vi "UI_(08A)_Prepare_loaded_data_playback.vi"(4 "Timeline max, s":dbl, 6 "error in (no error)":errorcluster, 8 "Timeline min, s":dbl, 9 "Settings cluster in":T1={"Defaults"={"Default User"=0.0, "VISA Resource Name "=""}, "Recording and saving"={"Researcher name"="", "Name prefix"="", "Data post-processing"={"Filter type"=enum."Savitzky-Golay", "Length"=31, "Order"=3}, "Stop at"=0.0, "\"Stop at\" enabled"=FALSE, "Default save folder path"=path "", "Acquisition FPS"=enum."Max"}, "Geometry"={"Cage diameter, mm"=0, "Starting angle MIDFIELD"=0, "Starting angle BORDER"=0, "Radius, mm CENTER"=0, "Radius, mm MIDFIELD"=0, "N segments MIDFIELD"=0, "N segments BORDER"=0, "R-gap, mm"=0.0, "Bridge swap"=FALSE, "Bridge H. offset"=0.0, "Bridge V. offset"=0.0, "Twisted neck"=FALSE, "Alt. magn. orientation"=FALSE, "Sensor board size"=enum."Small"}, "IO parameters"={"IO general config."=0, "IO 1 configuration"=0, "IO 2 configuration"=0, "IO 3 configuration"=0, "IO 4 configuration"=0, "Activate ext. RS-232"=0, "IO inversion config."=0, "Sync capability"=1}, "Stimulus presets array"=[{"Event type"=0, "Dur., s"=0.0, "Stim., s"=0.0, "TTL out N"=1, "Set/Clear"=FALSE, "Stim. has been set"=FALSE}, {"Event type"=0, "Dur., s"=0.0, "Stim., s"=0.0, "TTL out N"=1, "Set/Clear"=FALSE, "Stim. has been set"=FALSE}, {"Event type"=0, "Dur., s"=0.0, "Stim., s"=0.0, "TTL out N"=1, "Set/Clear"=FALSE, "Stim. has been set"=FALSE}, {"Event type"=0, "Dur., s"=0.0, "Stim., s"=0.0, "TTL out N"=1, "Set/Clear"=FALSE, "Stim. has been set"=FALSE}, {"Event type"=0, "Dur., s"=0.0, "Stim., s"=0.0, "TTL out N"=1, "Set/Clear"=FALSE, "Stim. has been set"=FALSE}, {"Event type"=0, "Dur., s"=0.0, "Stim., s"=0.0, "TTL out N"=1, "Set/Clear"=FALSE, "Stim. has been set"=FALSE}, {"Event type"=0, "Dur., s"=0.0, "Stim., s"=0.0, "TTL out N"=1, "Set/Clear"=FALSE, "Stim. has been set"=FALSE}, {"Event type"=0, "Dur., s"=0.0, "Stim., s"=0.0, "TTL out N"=1, "Set/Clear"=FALSE, "Stim. has been set"=FALSE}, {"Event type"=0, "Dur., s"=0.0, "Stim., s"=0.0, "TTL out N"=1, "Set/Clear"=FALSE, "Stim. has been set"=FALSE}, {"Event type"=0, "Dur., s"=0.0, "Stim., s"=0.0, "TTL out N"=1, "Set/Clear"=FALSE, "Stim. has been set"=FALSE}, {"Event type"=0, "Dur., s"=0.0, "Stim., s"=0.0, "TTL out N"=1, "Set/Clear"=FALSE, "Stim. has been set"=FALSE}, {"Event type"=0, "Dur., s"=0.0, "Stim., s"=0.0, "TTL out N"=1, "Set/Clear"=FALSE, "Stim. has been set"=FALSE}, {"Event type"=0, "Dur., s"=0.0, "Stim., s"=0.0, "TTL out N"=1, "Set/Clear"=FALSE, "Stim. has been set"=FALSE}, {"Event type"=0, "Dur., s"=0.0, "Stim., s"=0.0, "TTL out N"=1, "Set/Clear"=FALSE, "Stim. has been set"=FALSE}], "Calibration parameters"={"Timing calibration sw/hw"=1.0, "True FPS"=80.0, "True frame time, s"=0.0125, "Disp. calibration info"=[]}, "Settings loaded OK"=FALSE} {"Calibration parameters"."True frame time, s" format="%.10g"; "Calibration parameters"."Disp. calibration info"."Speed, µl per ms" format="%.3g"; "Calibration parameters"."True FPS" format="%.10g"; "Calibration parameters"."Timing calibration sw/hw" format="%.10g"; "Stimulus presets array"."Event type" items=["Stay for N seconds"]; "Stimulus presets array"."TTL out N" items=["1"=1, "2"=2, "1+2"=3]; "Recording and saving"."Data post-processing"."Order" min=3 max=11 step=2; "Recording and saving"."Data post-processing"."Length" min=5 max=301 step=2; "Geometry"."Cage diameter, mm" scale=0.0..340.0}, 10 "All references in":T11) -> (0 "error out":errorcluster, 2 "Settings cluster out":T1={"Defaults"={"Default User"=0.0, "VISA Resource Name "=""}, "Recording and saving"={"Researcher name"="", "Name prefix"="", "Data post-processing"={"Filter type"=enum."Savitzky-Golay", "Length"=31, "Order"=3}, "Stop at"=0.0, "\"Stop at\" enabled"=FALSE, "Default save folder path"=path "", "Acquisition FPS"=enum."Max"}, "Geometry"={"Cage diameter, mm"=0, "Starting angle MIDFIELD"=0, "Starting angle BORDER"=0, "Radius, mm CENTER"=0, "Radius, mm MIDFIELD"=0, "N segments MIDFIELD"=0, "N segments BORDER"=0, "R-gap, mm"=0.0, "Bridge swap"=FALSE, "Bridge H. offset"=0.0, "Bridge V. offset"=0.0, "Twisted neck"=FALSE, "Alt. magn. orientation"=FALSE, "Sensor board size"=enum."Small"}, "IO parameters"={"IO general config."=0, "IO 1 configuration"=0, "IO 2 configuration"=0, "IO 3 configuration"=0, "IO 4 configuration"=0, "Activate ext. RS-232"=0, "IO inversion config."=0, "Sync capability"=1}, "Stimulus presets array"=[{"Event type"=0, "Dur., s"=0.0, "Stim., s"=0.0, "TTL out N"=1, "Set/Clear"=FALSE, "Stim. has been set"=FALSE}, {"Event type"=0, "Dur., s"=0.0, "Stim., s"=0.0, "TTL out N"=1, "Set/Clear"=FALSE, "Stim. has been set"=FALSE}, {"Event type"=0, "Dur., s"=0.0, "Stim., s"=0.0, "TTL out N"=1, "Set/Clear"=FALSE, "Stim. has been set"=FALSE}, {"Event type"=0, "Dur., s"=0.0, "Stim., s"=0.0, "TTL out N"=1, "Set/Clear"=FALSE, "Stim. has been set"=FALSE}, {"Event type"=0, "Dur., s"=0.0, "Stim., s"=0.0, "TTL out N"=1, "Set/Clear"=FALSE, "Stim. has been set"=FALSE}, {"Event type"=0, "Dur., s"=0.0, "Stim., s"=0.0, "TTL out N"=1, "Set/Clear"=FALSE, "Stim. has been set"=FALSE}, {"Event type"=0, "Dur., s"=0.0, "Stim., s"=0.0, "TTL out N"=1, "Set/Clear"=FALSE, "Stim. has been set"=FALSE}, {"Event type"=0, "Dur., s"=0.0, "Stim., s"=0.0, "TTL out N"=1, "Set/Clear"=FALSE, "Stim. has been set"=FALSE}, {"Event type"=0, "Dur., s"=0.0, "Stim., s"=0.0, "TTL out N"=1, "Set/Clear"=FALSE, "Stim. has been set"=FALSE}, {"Event type"=0, "Dur., s"=0.0, "Stim., s"=0.0, "TTL out N"=1, "Set/Clear"=FALSE, "Stim. has been set"=FALSE}, {"Event type"=0, "Dur., s"=0.0, "Stim., s"=0.0, "TTL out N"=1, "Set/Clear"=FALSE, "Stim. has been set"=FALSE}, {"Event type"=0, "Dur., s"=0.0, "Stim., s"=0.0, "TTL out N"=1, "Set/Clear"=FALSE, "Stim. has been set"=FALSE}, {"Event type"=0, "Dur., s"=0.0, "Stim., s"=0.0, "TTL out N"=1, "Set/Clear"=FALSE, "Stim. has been set"=FALSE}, {"Event type"=0, "Dur., s"=0.0, "Stim., s"=0.0, "TTL out N"=1, "Set/Clear"=FALSE, "Stim. has been set"=FALSE}], "Calibration parameters"={"Timing calibration sw/hw"=1.0, "True FPS"=80.0, "True frame time, s"=0.0125, "Disp. calibration info"=[]}, "Settings loaded OK"=FALSE} {"Calibration parameters"."True frame time, s" format="%.10g"; "Calibration parameters"."Disp. calibration info"."Speed, µl per ms" format="%.3g"; "Calibration parameters"."True FPS" format="%.10g"; "Calibration parameters"."Timing calibration sw/hw" format="%.10g"; "Stimulus presets array"."Event type" items=["Stay for N seconds"]; "Stimulus presets array"."TTL out N" items=["1"=1, "2"=2, "1+2"=3]; "Recording and saving"."Data post-processing"."Order" min=3 max=11 step=2; "Recording and saving"."Data post-processing"."Length" min=5 max=301 step=2; "Geometry"."Cage diameter, mm" scale=0.0..340.0}, 3 "All references out":T11)   [LabVIEW 2018, in "Tracker.lvlib"]
uses:
  Tracker.lvlib
  Controls/CTL_All_References.ctl
  Controls/CTL_Controls_References.ctl
  Controls/CTL_Indicators_References.ctl
  Controls/CTL_Panes_and_VIs_References.ctl
  Controls/CTL_Histogram_Properties.ctl
  <vilib>/Utility/miscctls.llb/LVRangeTypeDef.ctl
  Controls/CTL_Settings_cluster.ctl
  Controls/CTL_Filter_selector.ctl
  Controls/CTL_Acquisition_speed_selector.ctl
  Controls/CTL_Segmented_plot_parameters.ctl
  Controls/CTL_IO_params_cluster.ctl
  Controls/CTL_Single_stimulus_setting.ctl
  Controls/CTL_Calibration_parameters.ctl
  Controls/CTL_Dispenser_calibration_info.ctl
  <vilib>/Utility/error.llb/Error Cluster From Error Code.vi
  <vilib>/ErrorRing/Error Ring.xnode
panel:
  in  "Histogram initialization cluster":T9={"X Scale.Range"={"Minimum"=0.0, "Maximum"=13.0, "Increment"=1.0, "Minor Increment"=1.0, "Start"=0.0}, "Caption.Text"="Zone preference (normalized)", "X Scale.Offset and Multiplier:Multiplier"=1.0, "X Scale.Offset and Multiplier:Offset"=0.0, "X Scale.Scale Fit"=2, "X Scale.Display Format:Precision"=0, "Y Scale.Mapping Mode"=0, "Zones preference empty initialized array"=[0, 0, 0, 0, 0, 0, 0, 0, 0, 0, 0, 0, 0, 0], "Plot.Fill/Point Color"=15790320}
  out "Panes references":T14
  out "Controls references params":string[][](array[string])
  out "Indicators references params":string[][](array[string])
  out "Indicators references":T13
  out "Controls references":T12
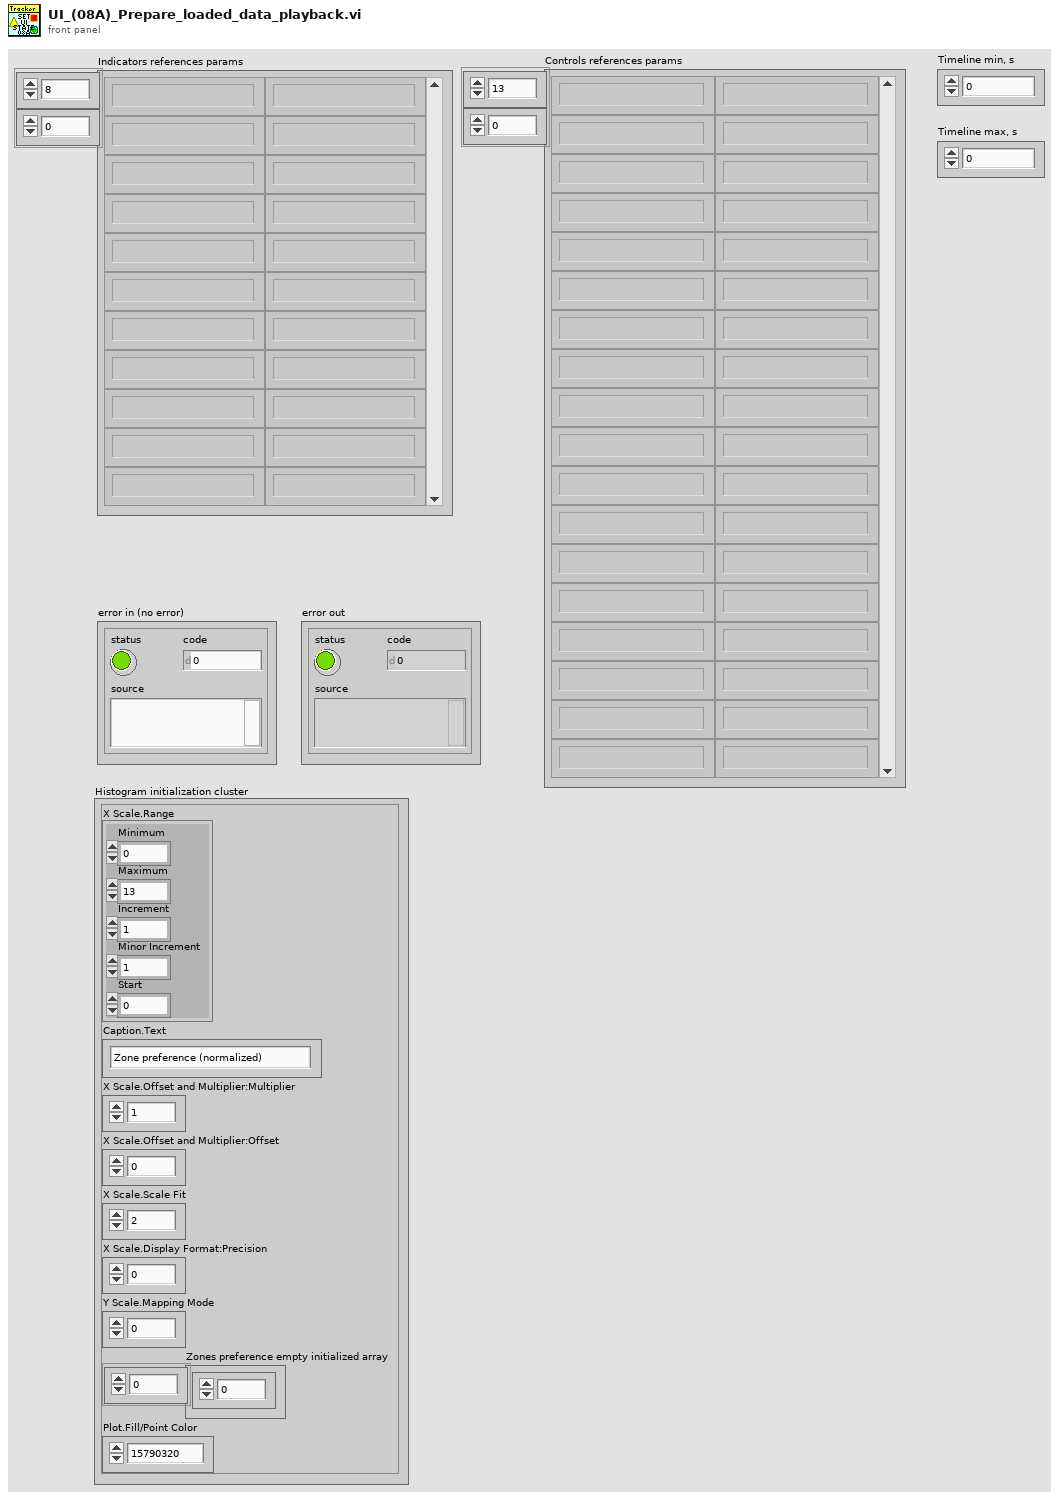
[diagram p1: front panel]
types:
  T1 = typedef "Tracker.lvlib/CTL_Settings_cluster.ctl" = cluster{"Defaults":cluster{"Default User":dbl, "VISA Resource Name ":string}, "Recording and saving":cluster{"Researcher name":string, "Name prefix":string, "Data post-processing":T2, "Stop at":dbl, "\"Stop at\" enabled":bool, "Default save folder path":path, "Acquisition FPS":T3}, "Geometry":T4, "IO parameters":T5, "Stimulus presets array":T6[], "Calibration parameters":T7, "Settings loaded OK":bool}
  T2 = typedef "Tracker.lvlib/CTL_Filter_selector.ctl" = cluster{"Filter type":enum16{"None", "Savitzky-Golay"}, "Length":i32, "Order":i32}
  T3 = typedef "Tracker.lvlib/CTL_Acquisition_speed_selector.ctl" = enum16{"Max", "Optimal", "Eco"}
  T4 = typedef "Tracker.lvlib/CTL_Segmented_plot_parameters.ctl" = cluster{"Cage diameter, mm":u16, "Starting angle MIDFIELD":i16, "Starting angle BORDER":i16, "Radius, mm CENTER":u16, "Radius, mm MIDFIELD":u16, "N segments MIDFIELD":u8, "N segments BORDER":u8, "R-gap, mm":sgl, "Bridge swap":bool, "Bridge H. offset":sgl, "Bridge V. offset":sgl, "Twisted neck":bool, "Alt. magn. orientation":bool, "Sensor board size":enum16{"Small", "Large"}}
  T5 = typedef "Tracker.lvlib/CTL_IO_params_cluster.ctl" = cluster{"IO general config.":u16, "IO 1 configuration":u16, "IO 2 configuration":u16, "IO 3 configuration":u16, "IO 4 configuration":u16, "Activate ext. RS-232":u16, "IO inversion config.":u16, "Sync capability":u8}
  T6 = typedef "Tracker.lvlib/CTL_Single_stimulus_setting.ctl" = cluster{"Event type":u16, "Dur., s":sgl, "Stim., s":sgl, "TTL out N":u16, "Set/Clear":bool, "Stim. has been set":bool}
  T7 = typedef "Tracker.lvlib/CTL_Calibration_parameters.ctl" = cluster{"Timing calibration sw/hw":dbl, "True FPS":dbl, "True frame time, s":dbl, "Disp. calibration info":T8}
  T8 = typedef "Tracker.lvlib/CTL_Dispenser_calibration_info.ctl" = cluster{"Channel":u8, "Speed, µl per ms":dbl}[]
  T9 = typedef "Tracker.lvlib/CTL_Histogram_Properties.ctl" = cluster{"X Scale.Range":T10, "Caption.Text":string, "X Scale.Offset and Multiplier:Multiplier":dbl, "X Scale.Offset and Multiplier:Offset":dbl, "X Scale.Scale Fit":u8, "X Scale.Display Format:Precision":u8, "Y Scale.Mapping Mode":u8, "Zones preference empty initialized array":i32[], "Plot.Fill/Point Color":u32}
  T10 = typedef "LVRangeTypeDef.ctl" = cluster{"Minimum":dbl, "Maximum":dbl, "Increment":dbl, "Minor Increment":dbl, "Start":dbl}
  T11 = typedef "Tracker.lvlib/CTL_All_References.ctl" = cluster{"Controls references":T12, "Indicators references":T13, "Service references":T14}
  T12 = typedef "Tracker.lvlib/CTL_Controls_References.ctl" = cluster{"Check HW connection":refnum<vi>, "Save settings":refnum<vi>, "Reset zones":refnum<vi>, "Reset stimuli":refnum<vi>, "Record/Stop":refnum<vi>, "Reset barplot":refnum<vi>, "Multiplyer of chart RX":refnum<vi>, "Show zones":refnum<vi>, "Show magnets":refnum<vi>, "Show heatmap":refnum<vi>, "Show full track":refnum<vi>, "Open File":refnum<vi>, "Play/Pause":refnum<vi>, "Trace, s":refnum<vi>, "Playback speed":refnum<vi>, "Timeline":refnum<vi>, "By Zone stim. setup":refnum<vi>, "Set/Rec and Analyse Tab":refnum<vi>, "Cage radial segmentation":refnum<vi>, "Set IO config":refnum<vi>, "Rainbow (time)":refnum<vi>, "Rainbow (speed)":refnum<vi>}
  T13 = typedef "Tracker.lvlib/CTL_Indicators_References.ctl" = cluster{"HW info":refnum<vi>, "Port":refnum<vi>, "Ready":refnum<vi>, "IO status indicator":refnum<vi>, "Current Time":refnum<vi>, "Record timestamp":refnum<vi>, "Mouse speed":refnum<vi>, "Mouse speed, mm/s":refnum<vi>, "Running, perc. of time":refnum<vi>, "Histograms":refnum<vi>, "Cage size":refnum<vi>}
  T14 = typedef "Tracker.lvlib/CTL_Panes_and_VIs_References.ctl" = cluster{"Pane":refnum<vi>, "This VI":refnum<vi>, "Menu":refnum<k9>}
  T15 = enum8{"Enabled", "Disabled", "Disabled and Grayed Out"}
  T16 = cluster{"Slider":dbl, "Slider":dbl, "Slider":dbl}
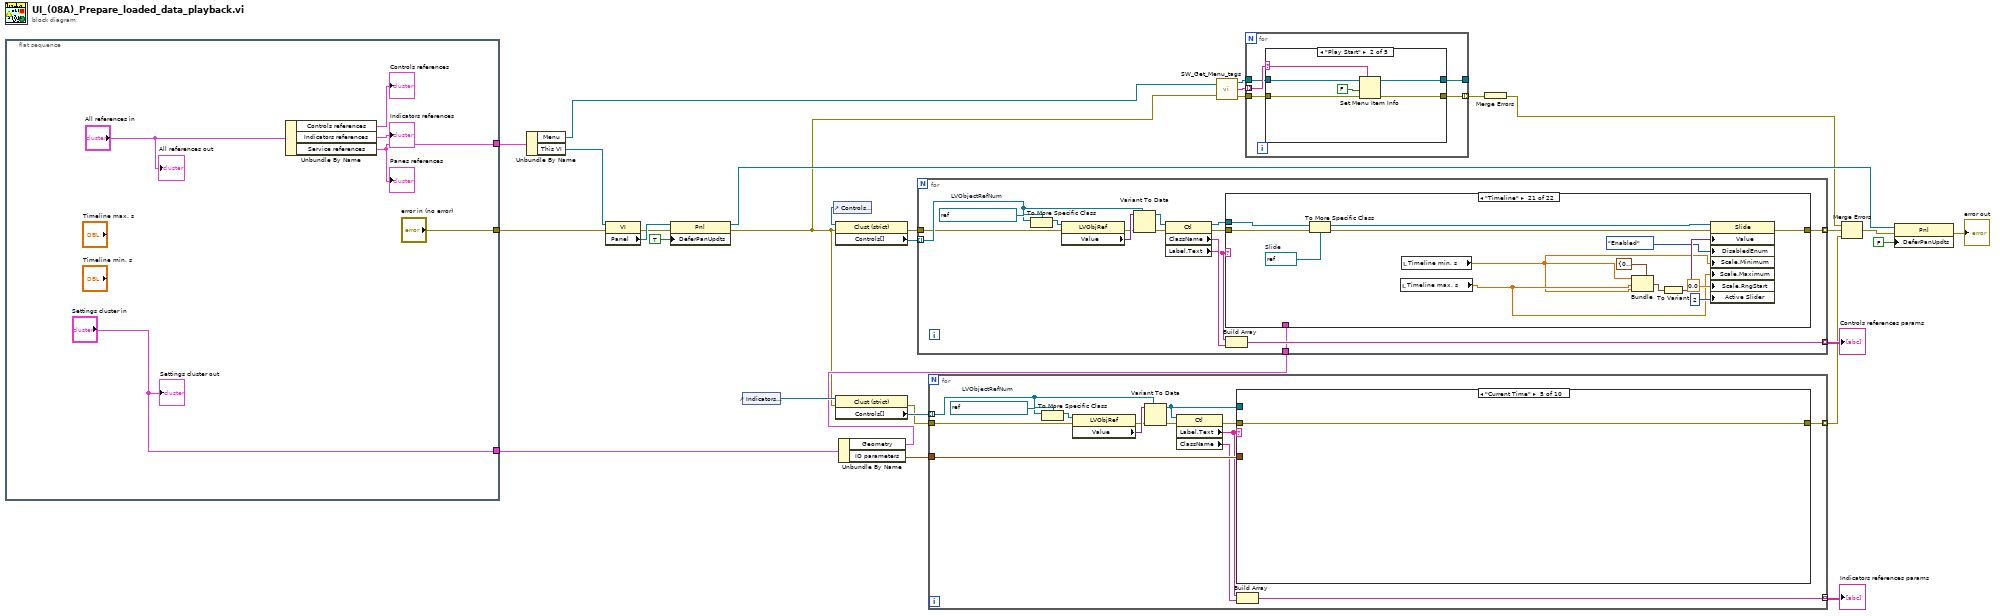
[diagram p0: block diagram]
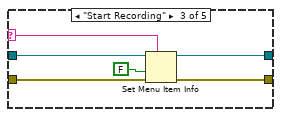
[diagram p3: hidden frame]
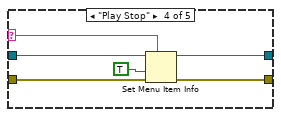
[diagram p4: hidden frame]
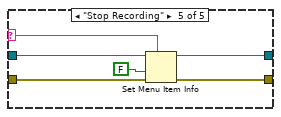
[diagram p5: hidden frame]
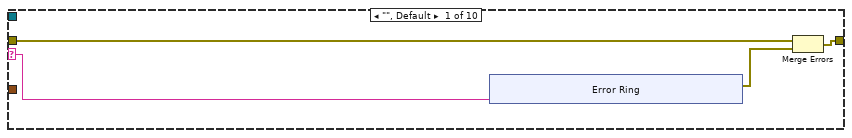
[diagram p6: hidden frame]
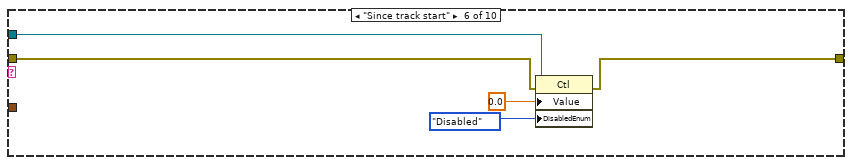
[diagram p10: hidden frame]
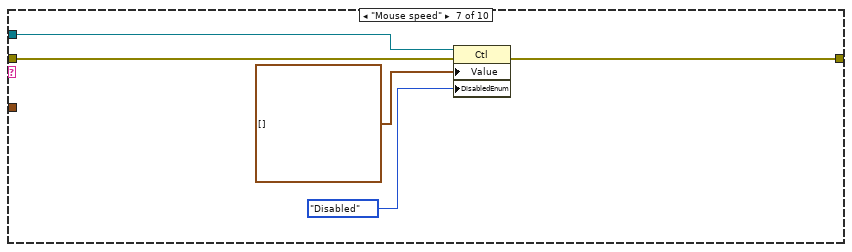
[diagram p11: hidden frame]
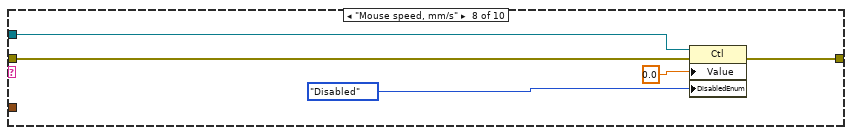
[diagram p12: hidden frame]
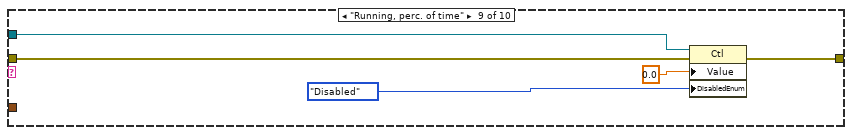
[diagram p13: hidden frame]
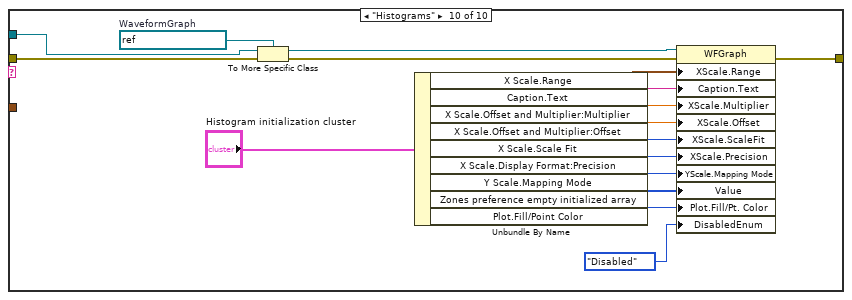
[diagram p14: hidden frame]
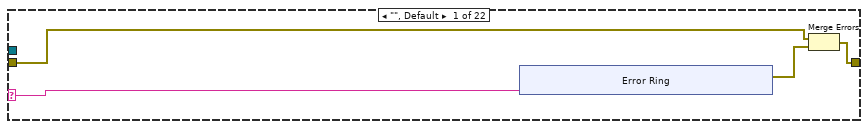
[diagram p15: hidden frame]
diagram:
  n1 = flat-sequence {
    tunnel: [w33] -> w24
    tunnel: ["Settings cluster in"] -> w11
    tunnel: ["error in (no error)"] -> w9
    frame #0 {
      n2 = Unbundle By Name("All references in") -> ("Controls references"=→"Controls references":T12, "Indicators references"=→"Indicators references":T13, "Service references"=w33:T14)
      "Panes references" <- w33
      "All references out" <- "All references in"
      "Settings cluster out" <- "Settings cluster in"
    }
  }
  n3 = Unbundle By Name(w24) -> ("Menu"=w3:refnum<k9>, "This VI"=w21:refnum<vi>)
  n4 = property class="VI"(reference=w21, error in=w9) -> (error out=w14:errorcluster, "Panel"=w23:refnum<vi>)  [unwired: 1 out]
  n5 = property class="Pnl"(reference=w23, error in=w14, "DeferPanUpdts"=TRUE ("Defer Panel Updates")) -> (reference out=w15:refnum<vi>, error out=w2:errorcluster)
  n6 = control-ref of="Indicators references"() -> (w27:refnum<vi>)
  n7 = control-ref of="Controls references"() -> (w29:refnum<vi>)
  n8 = property class="Clust (strict)"(reference=w29, error in=w2) -> (error out=w20:errorcluster, "Controls[]"=w30:refnum<vi>[])  [unwired: 1 out]
  n9 = property class="Clust (strict)"(reference=w27, error in=w2) -> (error out=w19:errorcluster, "Controls[]"=w28:refnum<vi>[])  [unwired: 1 out]
  n10 = Unbundle By Name(w11) -> ("Geometry"=w8:T4, "IO parameters"=w10:T5)
  n11 = for {
    tunnel: w30 -> [w48] mode=indexing
    tunnel: [w45] -> w25 mode=indexing
    tunnel: w20 -> [w44]
    tunnel: [w40] -> w12 mode=indexing
    tunnel: w8 -> [w37]
    w50 = refnum<vi> refnum  # LVObjectRefNum
    n12 = To More Specific Class(target class=w50, reference=w48) -> (specific class reference=w51:refnum<vi>)  [unwired: 1 in, 1 out]
    n13 = property class="LVObjRef"(reference=w51, error in=w44) -> (error out=w43:errorcluster, "Value"=w49:variant)  [unwired: 1 out]
    n14 = Variant To Data(error in=w43, type=w48, Variant=w49) -> (data=w47:refnum<vi>, error out=w42:errorcluster)
    n15 = property class="Ctl"(reference=w47, error in=w42) -> (reference out=w38:refnum<vi>, error out=w39:errorcluster, "ClassName"=w46:string, "Label.Text"=w41:string)
    n16 = case shown="\"Timeline\"" w41 {
      selector: w41 -> [w52 _ _ _ _ _ _ _ _ _ _ _ _ _ _ _ _ _ _ _ _ _]
      tunnel: [w54 w63 w64 w65 w66 w67 w68 w69 w72 w80 w88 w96 w102 w103 w112 w118 w128 w129 w132 w140 w154 w160] -> w40
      tunnel: w39 -> [w55 w63 w64 w65 w66 w67 w68 w69 w74 w82 w90 w98 w102 w105 w114 w118 w128 w129 w134 w142 w156 w160]
      tunnel: w38 -> [_ _ _ _ _ _ _ _ w77 w85 w93 w101 _ w104 w117 w119 _ _ w137 w145 w159 _]
      tunnel: w37 -> [_ _ _ _ _ _ _ _ _ _ _ _ _ _ _ _ _ _ _ _ _ _]
      frame "", Default {
        n17 = xnode "Error Ring"("parameter 0"=w52) -> ("error out"=w53:errorcluster)
        n18 = Merge Errors(w55, w53) -> (w54:errorcluster)
      }
      frame "Cage radial segmentation" {
      }
      frame "Set/Rec and Analyse Tab" {
      }
      frame "Check HW connection" {
      }
      frame "Save settings" {
      }
      frame "Set IO config" {
      }
      frame "Reset zones" {
      }
      frame "Reset stimuli" {
      }
      frame "Record/Stop" {
        w76 = refnum<vi> refnum  # Boolean
        n19 = To More Specific Class(target class=w76, reference=w77, error in=w74) -> (specific class reference=w75:refnum<vi>, error out=w73:errorcluster)
        n20 = property class="Bool"(reference=w75, error in=w73, "Value"=FALSE, "DisabledEnum"=T15."Disabled and Grayed Out" ("Disabled")) -> (error out=w72:errorcluster)  [unwired: 1 out]
      }
      frame "Reset barplot" {
        w84 = refnum<vi> refnum  # Boolean
        n21 = To More Specific Class(target class=w84, reference=w85, error in=w82) -> (specific class reference=w83:refnum<vi>, error out=w81:errorcluster)
        n22 = property class="Bool"(reference=w83, error in=w81, "Value"=FALSE, "DisabledEnum"=T15."Enabled" ("Disabled")) -> (error out=w80:errorcluster)  [unwired: 1 out]
      }
      frame "Multiplyer of chart RX" {
        w92 = refnum<vi> refnum  # Slide
        n23 = To More Specific Class(target class=w92, reference=w93, error in=w90) -> (specific class reference=w91:refnum<vi>, error out=w89:errorcluster)
        n24 = property class="Slide"(reference=w91, error in=w89, "Value"=u8 1, "DisabledEnum"=T15."Enabled" ("Disabled")) -> (error out=w88:errorcluster)  [unwired: 1 out]
      }
      frame "Show zones" {
        w100 = refnum<vi> refnum  # Boolean
        n25 = To More Specific Class(target class=w100, reference=w101, error in=w98) -> (specific class reference=w99:refnum<vi>, error out=w97:errorcluster)
        n26 = property class="Bool"(reference=w99, error in=w97, "Value"=TRUE, "DisabledEnum"=T15."Enabled" ("Disabled")) -> (error out=w96:errorcluster)  [unwired: 1 out]
      }
      frame "Show magnets" {
      }
      frame "Rainbow (speed)", "Rainbow (time)" {
        w106 = refnum<vi> refnum  # Boolean
        n27 = To More Specific Class(target class=w106, reference=w104, error in=w105) -> (specific class reference=w108:refnum<vi>, error out=w109:errorcluster)
        n28 = property class="Bool"(reference=w108, error in=w109, "DisabledEnum"=T15."Enabled" ("Disabled")) -> (error out=w103:errorcluster)  [unwired: 1 out]
      }
      frame "Show heatmap" {
        w116 = refnum<vi> refnum  # Boolean
        n29 = To More Specific Class(target class=w116, reference=w117, error in=w114) -> (specific class reference=w115:refnum<vi>, error out=w113:errorcluster)
        n30 = property class="Bool"(reference=w115, error in=w113, "Value"=FALSE, "DisabledEnum"=T15."Disabled and Grayed Out" ("Disabled")) -> (error out=w112:errorcluster)  [unwired: 1 out]
      }
      frame "Show full track" {
        n31 = disable-structure shown="Disabled" {
          disable-tunnel: w119 -> [w127 _]
          disable-tunnel: _ -> [w124 _]
          disable-tunnel: [w122 _] -> _
          frame Disabled {
            w126 = refnum<vi> refnum  # Boolean
            n32 = To More Specific Class(target class=w126, reference=w127, error in=w124) -> (specific class reference=w125:refnum<vi>, error out=w123:errorcluster)
            n33 = property class="Bool"(reference=w125, error in=w123, "Value"=FALSE, "DisabledEnum"=T15."Disabled and Grayed Out" ("Disabled")) -> (error out=w122:errorcluster)  [unwired: 1 out]
          }
          frame Enabled {
          }
        }
      }
      frame "Open File" {
      }
      frame "Play/Pause" {
      }
      frame "Trace, s" {
        w136 = refnum<vi> refnum  # Slide
        n34 = To More Specific Class(target class=w136, reference=w137, error in=w134) -> (specific class reference=w135:refnum<vi>, error out=w133:errorcluster)
        n35 = property class="Slide"(reference=w135, error in=w133, "Value"=u8 5, "DisabledEnum"=T15."Enabled" ("Disabled")) -> (error out=w132:errorcluster)  [unwired: 1 out]
      }
      frame "Playback speed" {
        w144 = refnum<vi> refnum  # Ring
        n36 = To More Specific Class(target class=w144, reference=w145, error in=w142) -> (specific class reference=w143:refnum<vi>, error out=w141:errorcluster)
        n37 = property class="Ring"(reference=w143, error in=w141, "Value"=u8 3, "DisabledEnum"=T15."Disabled and Grayed Out" ("Disabled")) -> (error out=w140:errorcluster)  [unwired: 1 out]
      }
      frame "Timeline" {
        w158 = refnum<vi> refnum  # Slide
        n38 = To More Specific Class(target class=w158, reference=w159, error in=w156) -> (specific class reference=w157:refnum<vi>, error out=w155:errorcluster)
        n39 = local read "Timeline max, s"() -> (w147:dbl)
        n40 = local read "Timeline min, s"() -> (w146:dbl)
        n41 = Bundle(cluster=T16 {"Slider"=0.0, "Slider"=0.0, "Slider"=0.0} ("Timeline"), "Slider"=w146, "Slider"=w147, "Slider"=w146) -> (w152:T16)
        n42 = To Variant(anything=w152) -> (Variant=w151:variant)
        n43 = property class="Slide"(reference=w157, error in=w155, "Value"=w151, "DisabledEnum"=T15."Enabled" ("Disabled"), "Scale.Minimum"=w146, "Scale.Maximum"=w147, "Scale.RngStart"=0.0 ("Scale.Range:Start"), "Active Slider"=2) -> (error out=w154:errorcluster)  [unwired: 1 out]
      }
      frame "By Zone stim. setup" {
      }
    }
    n44 = Build Array(w41, w46) -> (w45:string[])
  }
  "Controls references params" <- w25
  n45 = for {
    tunnel: w28 -> [w171] mode=indexing
    tunnel: [w161] -> w26 mode=indexing
    tunnel: w19 -> [w169]
    tunnel: [w165] -> w18 mode=indexing
    tunnel: w10 -> [w164]
    w173 = refnum<vi> refnum  # LVObjectRefNum
    n46 = To More Specific Class(target class=w173, reference=w171) -> (specific class reference=w174:refnum<vi>)  [unwired: 1 in, 1 out]
    n47 = property class="LVObjRef"(reference=w174, error in=w169) -> (error out=w168:errorcluster, "Value"=w172:variant)  [unwired: 1 out]
    n48 = Variant To Data(error in=w168, type=w171, Variant=w172) -> (data=w170:refnum<vi>, error out=w167:errorcluster)
    n49 = property class="Ctl"(reference=w170, error in=w167) -> (error out=w166:errorcluster, "Label.Text"=w163:string, "ClassName"=w162:string)  [unwired: 1 out]
    n50 = case shown="\"Current Time\"" w163 {
      selector: w163 -> [w175 _ _ _ _ _ _ _ _ _]
      tunnel: w170 -> [_ _ _ _ _ w190 w199 w204 w209 w226]
      tunnel: w166 -> [w178 w186 w187 w188 w189 w192 w198 w203 w208 w212]
      tunnel: [w177 w186 w187 w188 w189 w191 w197 w202 w207 w225] -> w165
      tunnel: w164 -> [_ _ _ _ _ _ _ _ _ _]
      frame "", Default {
        n51 = xnode "Error Ring"("parameter 0"=w175) -> ("error out"=w176:errorcluster)
        n52 = Merge Errors(w178, w176) -> (w177:errorcluster)
      }
      frame "Cage size", "HW info", "Port" {
      }
      frame "Ready" {
      }
      frame "IO status indicator" {
      }
      frame "Current Time" {
      }
      frame "Since track start" {
        n53 = property class="Ctl"(reference=w190, error in=w192, "Value"=0.0, "DisabledEnum"=T15."Disabled" ("Disabled")) -> (error out=w191:errorcluster)  [unwired: 1 out]
      }
      frame "Mouse speed" {
        n54 = property class="Ctl"(reference=w199, error in=w198, "Value"=waveform(dbl)[] [] ("History Data"), "DisabledEnum"=T15."Disabled" ("Disabled")) -> (error out=w197:errorcluster)  [unwired: 1 out]
      }
      frame "Mouse speed, mm/s" {
        n55 = property class="Ctl"(reference=w204, error in=w203, "Value"=0.0, "DisabledEnum"=T15."Disabled" ("Disabled")) -> (error out=w202:errorcluster)  [unwired: 1 out]
      }
      frame "Running, perc. of time" {
        n56 = property class="Ctl"(reference=w209, error in=w208, "Value"=0.0, "DisabledEnum"=T15."Disabled" ("Disabled")) -> (error out=w207:errorcluster)  [unwired: 1 out]
      }
      frame "Histograms" {
        w223 = refnum<vi> refnum  # WaveformGraph
        n57 = To More Specific Class(target class=w223, reference=w226, error in=w212) -> (specific class reference=w224:refnum<vi>, error out=w211:errorcluster)
        n58 = Unbundle By Name("Histogram initialization cluster") -> ("X Scale.Range"=w221:T10, "Caption.Text"=w220:string, "X Scale.Offset and Multiplier:Multiplier"=w219:dbl, "X Scale.Offset and Multiplier:Offset"=w218:dbl, "X Scale.Scale Fit"=w217:u8, "X Scale.Display Format:Precision"=w216:u8, "Y Scale.Mapping Mode"=w215:u8, "Zones preference empty initialized array"=w214:i32[], "Plot.Fill/Point Color"=w213:u32)
        n59 = property class="WFGraph"(reference=w224, error in=w211, "XScale.Range"=w221, "Caption.Text"=w220, "XScale.Multiplier"=w219, "XScale.Offset"=w218, "XScale.ScaleFit"=w217, "XScale.Precision"=w216, "YScale.Mapping Mode"=w215, "Value"=w214, "Plot.Fill/Pt. Color"=w213, "DisabledEnum"=T15."Disabled" ("Disabled")) -> (error out=w225:errorcluster)  [unwired: 1 out]
      }
    }
    n60 = Build Array(w163, w162) -> (w161:string[])
  }
  "Indicators references params" <- w26
  n61 = call "SW_Get_Menu_tags.vi"("Menu ref in"=w3, "error in (no error)"=w2) -> ("Menu ref out"=w5:refnum<k9>, "(Sub)menu tags"=w7:string[], "error out"=w6:errorcluster)
  n62 = for {
    tunnel: w7 -> [w231] mode=indexing
    tunnel: w6 -> [w230]
    tunnel: [w229] -> w4 mode=indexing
    tunnel: [w228] -> _
    tunnel: w5 -> [w227]
    n63 = case shown="\"Play Start\"" w231 {
      selector: w231 -> [_ w239 w245 w251 w257]
      tunnel: w230 -> [w233 w237 w243 w249 w255]
      tunnel: [w233 w236 w242 w248 w254] -> w229
      tunnel: [w232 w235 w241 w247 w253] -> w228
      tunnel: w227 -> [w232 w234 w240 w246 w252]
      frame "", Default {
      }
      frame "Play Start" {
        n64 = Set Menu Item Info(7:w239, 8:w237, 9:FALSE ("enabled"), 11:w234) -> (0:w236:errorcluster, 3:w235:refnum<k9>)  [unwired: 3 in]
      }
      frame "Start Recording" {
        n65 = Set Menu Item Info(7:w245, 8:w243, 9:FALSE ("enabled"), 11:w240) -> (0:w242:errorcluster, 3:w241:refnum<k9>)  [unwired: 3 in]
      }
      frame "Play Stop" {
        n66 = Set Menu Item Info(7:w251, 8:w249, 9:TRUE ("enabled"), 11:w246) -> (0:w248:errorcluster, 3:w247:refnum<k9>)  [unwired: 3 in]
      }
      frame "Stop Recording" {
        n67 = Set Menu Item Info(7:w257, 8:w255, 9:FALSE ("enabled"), 11:w252) -> (0:w254:errorcluster, 3:w253:refnum<k9>)  [unwired: 3 in]
      }
    }
  }
  n68 = Merge Errors(w4) -> (w1:errorcluster)
  n69 = Merge Errors(w1, w12, w18) -> (w17:errorcluster)
  n70 = property class="Pnl"(reference=w15, error in=w17, "DeferPanUpdts"=FALSE ("Defer Panel Updates")) -> (error out=→"error out":errorcluster)  [unwired: 1 out]
